vi "XY Graph Modern.vi"() -> ()   [LabVIEW 2021, in "XY Graph Add-Ons.lvlib"]
uses:
  XY Graph Add-Ons.lvlib
  XY Graph Plot Data.ctl
panel:
  out "XY Graph":cluster{"X Array":dbl[], "Y Array":dbl[]}[](graph)
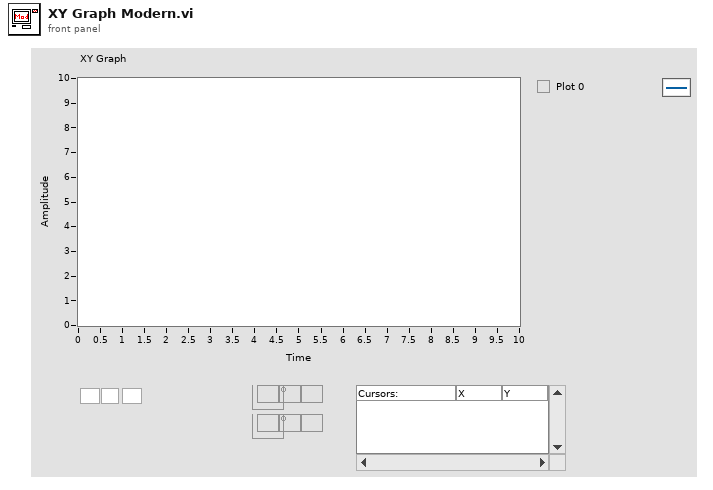
[diagram p1: front panel]
types:
  T1 = typedef "XY Graph Add-Ons.lvlib/XY Graph Plot Data.ctl" = cluster{"X Array":dbl[], "Y Array":dbl[]}
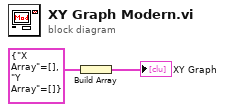
[diagram p0: block diagram]
diagram:
  n1 = Build Array(T1 {"X Array"=[], "Y Array"=[]} ("Plot")) -> (→"XY Graph":T1[])
